vi "remote.Build Init Request.vi"(6 "resource":string, 7 "connect timeout":dbl, 8 "error in (no error)":errorcluster, 9 "slsc type":T1, 10 "reservation access":i32, 11 "reservation group":string) -> (0 "error out":errorcluster, 3 "JSON Object out":refnum<class "JSON Object.lvclass">)   [LabVIEW 2016, in "SLSC Interfaces.lvlib" / "SLSC Interface.lvclass"]
uses:
  SLSC Interface Class/SLSC Interface.lvclass
  <vilib>/NI/JSON Support for LabVIEW/JSON Data Classes/JSON Helper/JSON Helper.lvclass
  <vilib>/NI/JSON Support for LabVIEW/JSON Data Classes/JSON Object/JSON Object.lvclass
  <vilib>/NI/JSON Support for LabVIEW/JSON Data Classes/JSON Object/Insert Key Value Pair (Single Numeric).vi
  <vilib>/NI/JSON Support for LabVIEW/JSON Data Classes/JSON Object/New JSON Object (Empty).vi
  <vilib>/NI/JSON Support for LabVIEW/JSON Data Classes/JSON Object/Insert Key Value Pair (Single String).vi
  SLSC Interface Class/slsc type.ctl
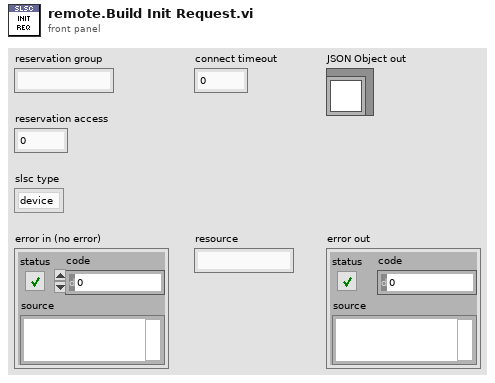
[diagram p1: front panel]
types:
  T1 = typedef "SLSC Interfaces.lvlib/SLSC Interface.lvclass/slsc type.ctl" = enum16{"device", "nvmem", "channel", "none"}
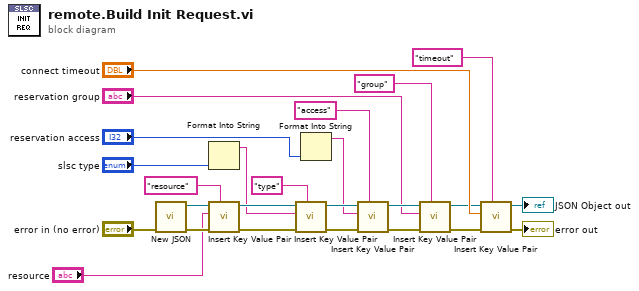
[diagram p0: block diagram]
diagram:
  n1 = call-poly <vilib>:"New JSON.vi"("error in (no error)"="error in (no error)") -> ("error out"=w18:errorcluster, "JSON Object out"=w12:refnum<class "JSON Object.lvclass">)  [unwired: 9 in]
  n2 = Format Into String("slsc type") -> (resulting string=w2:string)  [unwired: 3 in, 1 out]
  n3 = call-poly <vilib>:"Insert Key Value Pair.vi"("key"="resource" ("Name"), "error in (no error)"=w18, "value"="resource", "JSON Object in"=w12) -> ("error out"=w19:errorcluster, "JSON Object out"=w11:refnum<class "JSON Object.lvclass">)  [unwired: 5 in, 1 out]
  n4 = call-poly <vilib>:"Insert Key Value Pair.vi"("key"="type" ("Name"), "error in (no error)"=w19, "value"=w2, "JSON Object in"=w11) -> ("error out"=w22:errorcluster, "JSON Object out"=w10:refnum<class "JSON Object.lvclass">)  [unwired: 5 in, 1 out]
  n5 = Format Into String("reservation access") -> (resulting string=w3:string)  [unwired: 3 in, 1 out]
  n6 = call-poly <vilib>:"Insert Key Value Pair.vi"("key"="access" ("Name"), "error in (no error)"=w22, "value"=w3, "JSON Object in"=w10) -> ("error out"=w23:errorcluster, "JSON Object out"=w9:refnum<class "JSON Object.lvclass">)  [unwired: 5 in, 1 out]
  n7 = call-poly <vilib>:"Insert Key Value Pair.vi"("key"="group" ("Name"), "error in (no error)"=w23, "value"="reservation group", "JSON Object in"=w9) -> ("error out"=w24:errorcluster, "JSON Object out"=w13:refnum<class "JSON Object.lvclass">)  [unwired: 5 in, 1 out]
  n8 = call-poly <vilib>:"Insert Key Value Pair.vi"("key"="timeout" ("Name"), "error in (no error)"=w24, "value"="connect timeout", "JSON Object in"=w13) -> ("error out"=→"error out":errorcluster, "JSON Object out"=→"JSON Object out":refnum<class "JSON Object.lvclass">)  [unwired: 5 in, 1 out]
